vi "Read structures.vi"(9 "Diagram in":refnum<class "Diagram.lvclass">) -> (3 "Diagram out":refnum<class "Diagram.lvclass">, 4 "structures":refnum<class "Structure.lvclass">[](array[class]))   [LabVIEW 2014, in "Raspberry Pi Compatible Compiler for LabVIEW.lvlib" / "Diagram.lvclass"]
uses:
  Diagram.lvclass
  Structure/Structure.lvclass
  Diagram.lvclass/Diagram.ctl
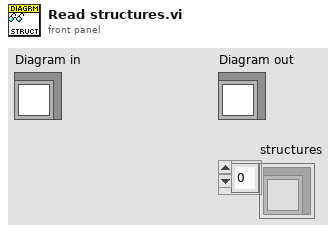
[diagram p1: front panel]
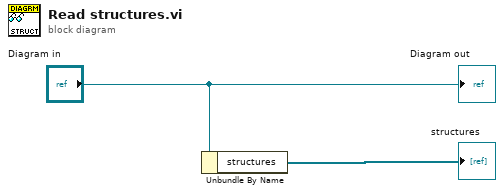
[diagram p0: block diagram]
diagram:
  n1 = Unbundle By Name("Diagram in") -> ("structures"=→"structures":refnum<class "Structure.lvclass">[])
  "Diagram out" <- "Diagram in"
